vi "LS330_Read_HEATERS.vi"(8 "error in (no error)":errorcluster, 10 "Heater":string(combo)="1", 11 "VISA Refnum in":refnum<visa-resource-name>) -> (0 "error out":errorcluster, 1 "Range":enum16{"Off", "Low", "Medium", "High"}(ring), 2 "Heater %":dbl, 3 "VISA Refnum out":refnum<visa-resource-name>)   [LabVIEW 2021]
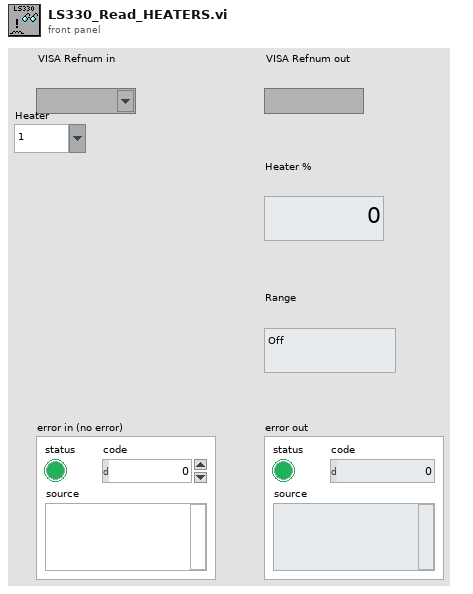
[diagram p1: front panel]
types:
  T1 = typedef "Heater_Range.ctl" = enum16{"Off", "Low", "Medium", "High"}
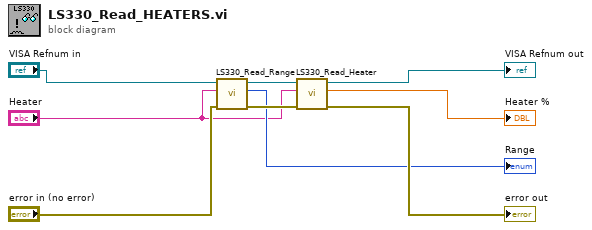
[diagram p0: block diagram]
diagram:
  n1 = call "LS330_Read_Range.vi"("error in"="error in (no error)", "Heater"="Heater", "VISA resource name"="VISA Refnum in") -> ("error out"=w6:errorcluster, "Range"=→"Range":T1, "VISA resource name out"=w5:refnum<visa-resource-name>)  [unwired: 6 in]
  n2 = call "LS330_Read_Heater.vi"("error in"=w6, "Heater"="Heater", "VISA resource name"=w5) -> ("error out"=→"error out":errorcluster, "Heater %"=→"Heater %":dbl, "VISA resource name out"=→"VISA Refnum out":refnum<visa-resource-name>)  [unwired: 6 in]
